vi "OPCUA.CreateConnectionString.vi"(10 "Server Port":u16, 11 "Server IP Address":string="localhost") -> (3 "concatenated string":string)   [LabVIEW 2013, in "OPC UA Client Shared.lvlib"]
uses:
  OPC UA Client Shared.lvlib
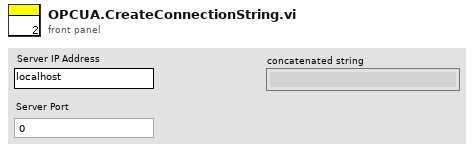
[diagram p1: front panel]
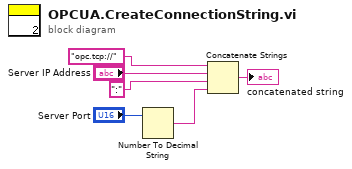
[diagram p0: block diagram]
diagram:
  n1 = Number To Decimal String(number="Server Port") -> (decimal integer string=w4:string)  [unwired: 1 in]
  n2 = Concatenate Strings("opc.tcp://", "Server IP Address", ":", w4) -> (→"concatenated string":string)
